vi "GearShift.vi"(8 "Gear2":bool=TRUE, 11 "Gear1":bool) -> ()   [LabVIEW 2018]
uses:
  <vilib>/Rock Robotics/WPI/Solenoid/WPI_SolenoidValue.ctl
  <vilib>/Rock Robotics/WPI/Solenoid/WPI_SolenoidSetEnum.vi
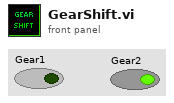
[diagram p1: front panel]
types:
  T1 = typedef "WPI_SolenoidValue.ctl" = enum16{"Off", "On", "Forward", "Reverse"}
  T2 = typedef "WPI_SolenoidDevRef.ctl" = cluster{"DevStatus":errorcluster, "Pneumatics Control Module":u8, "Forward Solenoid Channel":T3, "Reverse Solenoid Channel":T3}
  T3 = typedef "WPI_SolenoidChannel.ctl" = enum8{"Solenoid 0", "Solenoid 1", "Solenoid 2", "Solenoid 3", "Solenoid 4", "Solenoid 5", "Solenoid 6", "Solenoid 7", "Invalid"}
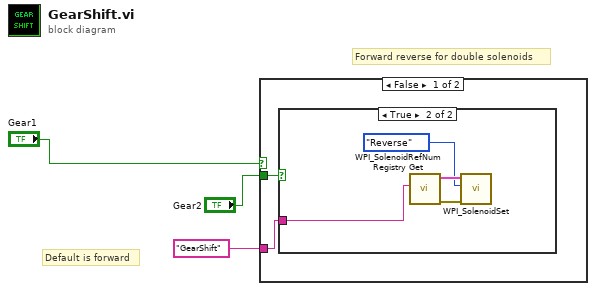
[diagram p0: block diagram]
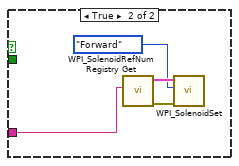
[diagram p3: hidden frame]
diagram:
  # "Default is forward"
  # "Forward reverse for double solenoids"
  n1 = case shown="False" "Gear1" {
    tunnel: "Gear2" -> [w5 _]
    tunnel: "GearShift" ("refnum name") -> [w4 w10]
    frame False {
      n2 = case shown="True" w5 {
        tunnel: w4 -> [_ w6]
        frame False {
        }
        frame True {
          n3 = call <vilib>:"WPI_SolenoidRefNum Registry Get.vi"("refnum name"=w6) -> ("error out"=w8:errorcluster, "SolenoidDevRef"=w9:T2)  [unwired: 9 in]
          n4 = call-poly <vilib>:"WPI_SolenoidSet.vi"("error in (no error)"=w8, "Value"=WPI_SolenoidValue."Reverse", "SolenoidDevRef"=w9) -> ()  [unwired: 7 in, 2 out]
        }
      }
    }
    frame True {
      n5 = call <vilib>:"WPI_SolenoidRefNum Registry Get.vi"("refnum name"=w10) -> ("error out"=w12:errorcluster, "SolenoidDevRef"=w13:T2)  [unwired: 9 in]
      n6 = call-poly <vilib>:"WPI_SolenoidSet.vi"("error in (no error)"=w12, "Value"=WPI_SolenoidValue."Forward", "SolenoidDevRef"=w13) -> ()  [unwired: 7 in, 2 out]
    }
  }
